vi "Set_epoch.vi"(1 "AnnéeRL":dbl, 2 "EPOCH_AFF":dbl format="%.1f") -> (0 "EPOCH_OUT":dbl format="%.1f")   [LabVIEW 2011]
panel:
  in  "y1950":bool
  in  "y2k":bool
  in  "act":bool
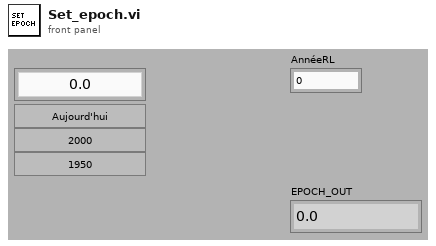
[diagram p1: front panel]
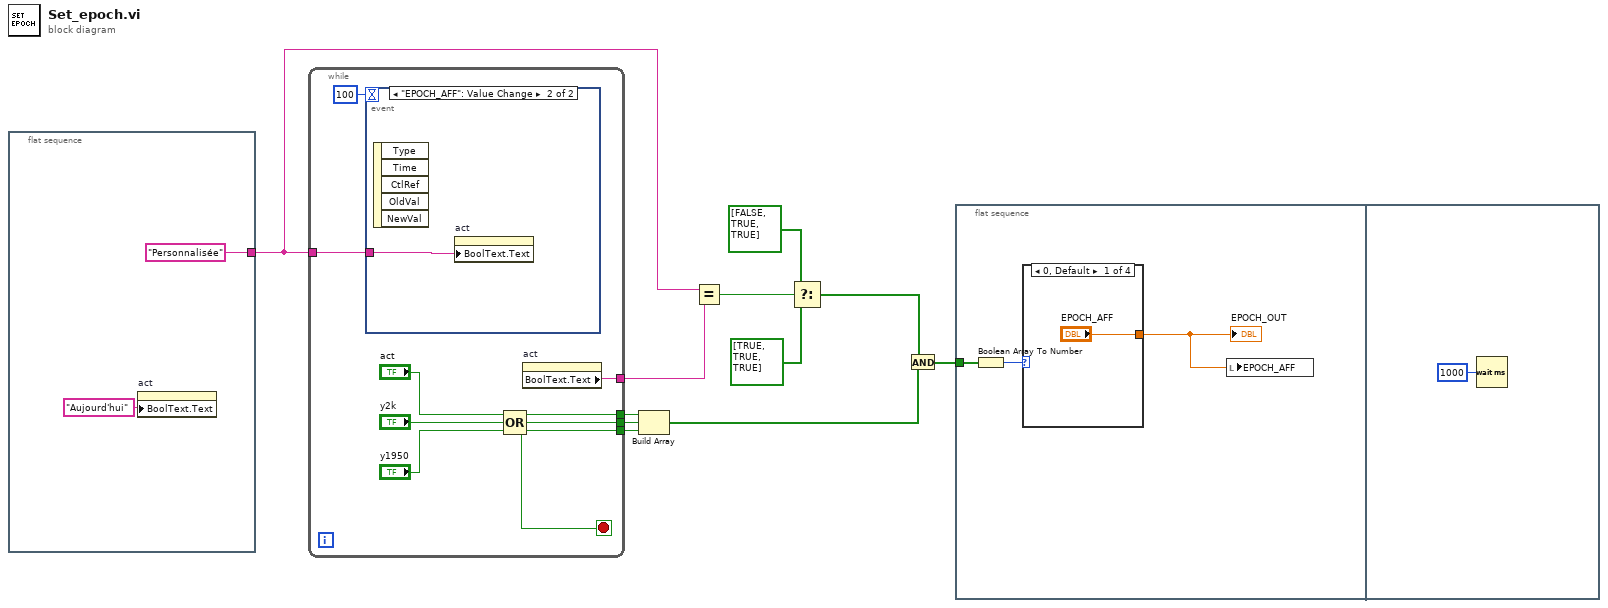
[diagram p0: block diagram]
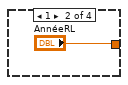
[diagram p2: hidden frame]
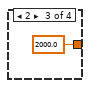
[diagram p3: hidden frame]
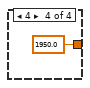
[diagram p4: hidden frame]
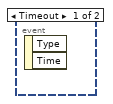
[diagram p5: hidden frame]
diagram:
  n1 = flat-sequence {
    tunnel: ["Personnalisée"] -> w2
    frame #0 {
      n2 = property on="act" class="Bool"("BoolText.Text"="Aujourd'hui" ("Boolean Text.Text")) -> ()  [unwired: 2 in, 2 out]
    }
  }
  n3 = while {
    tunnel: ["act"] -> w11
    tunnel: ["y2k"] -> w10
    tunnel: ["y1950"] -> w9
    tunnel: w2 -> [w15]
    tunnel: [w14] -> w1
    stop <- w20 stop-if-true
    n4 = event shown="[1] \"EPOCH_AFF\": Value Change" {
      selector: _ -> [_ _]
      dyn-events: _ -> [_ _]
      timeout: 100 -> [_ _]
      tunnel: w15 -> [_ w21]
      event Timeout {
        n5 = event-data() -> ()  [unwired: 1 in, 2 out]
      }
      event "EPOCH_AFF": Value Change {
        n6 = event-data() -> ()  [unwired: 1 in, 5 out]
        n7 = property on="act" class="Bool"("BoolText.Text"=w21) -> ()  [unwired: 2 in, 2 out]
      }
    }
    n8 = Compound Arithmetic op=OR("act", "y2k", "y1950") -> (w20:bool)
    n9 = property on="act" class="Bool"() -> ("BoolText.Text"=w14:string)  [unwired: 2 in, 2 out]
  }
  n10 = Build Array(w11, w10, w9) -> (w8:bool[])
  n11 = Equal?(x=w2, y=w1) -> (x = y?=w7:bool)
  n12 = Select(t=bool[] [FALSE, TRUE, TRUE], s=w7, f=bool[] [TRUE, TRUE, TRUE]) -> (s? t:f=w4:bool[])
  n13 = And(x=w4, y=w8) -> (x .and. y?=w3:bool[])
  n14 = flat-sequence {
    tunnel: w3 -> [w23]
    frame #0 {
      n15 = Boolean Array To Number(Boolean array=w23) -> (number=w24:u32)
      n16 = case shown="0, Default" w24 {
        tunnel: ["EPOCH_AFF" "AnnéeRL" 2000.0 ("AnnéeRL") 1950.0 ("AnnéeRL")] -> w22
        frame 0, Default {
        }
        frame 1 {
        }
        frame 2 {
        }
        frame 4 {
        }
      }
      "EPOCH_OUT" <- w22
      n17 = local write "EPOCH_AFF"(w22) -> ()
    }
    frame #1 {
      n18 = Wait (ms)(milliseconds to wait=u32 1000) -> ()  [unwired: 1 out]
    }
  }
